vi "Avoid obstacle button2.0.vi"() -> ()   [LabVIEW 2015]
uses:
  <userlib>/KNR OS 3.0 LabVIEW Toolkit/Type Definition/Resource.ctl
  <userlib>/KNR OS 3.0 LabVIEW Toolkit/Type Definition/DC Motor Port.ctl
  <userlib>/KNR OS 3.0 LabVIEW Toolkit/Type Definition/Ultrasonic Port Number.ctl
  <vilib>/myRIO/Common/Instrument Driver Framework/myRIO v1.0/UART/vis/myRIO v1.0 Close UART.vi
  <vilib>/myRIO/Common/Instrument Driver Framework/Utilities/vis/FPGA Ref Manager.vi
  <vilib>/myRIO/Common/Instrument Driver Framework/myRIO v1.0/myRIO v1.0 Reset FPGA.vi
  <vilib>/myRIO/Common/Instrument Driver Framework/myRIO v1.0/IRQ/vis/myRIO v1.0 IRQ Info FGV.vi
  <vilib>/myRIO/Common/Instrument Driver Framework/myRIO v1.0/IRQ/vis/myRIO v1.0 Timer IRQ Info FGV.vi
  <vilib>/myRIO/Common/Instrument Driver Framework/myRIO v1.0/IRQ/vis/myRIO v1.0 ISR Agent.vi
  <vilib>/myRIO/Instrument Drivers/Utilities/Utilities.lvlib
panel:
  in  "stop":bool
  in  "forward speed":dbl=5.8 format="%#_13g"
  out "Speed R 2":dbl=4.06
  out "Speed L 2":dbl=4.06
  in  "upper limit r":dbl=9.0
  in  "upper limit l":dbl=10.0
  in  "Speed":dbl=8.0
  in  "Distance":dbl=35.0
  in  "Kp":dbl=0.3
  in  "Reverse Encoder R":bool=TRUE
  in  "Reverse Encoder L":bool
  in  "Y":dbl
  in  "X":dbl=190.0
  out "Pos R":dbl=170.41358455446547
  out "Pos L":dbl=162.57741982327175
  out "Actual X":dbl=165.0804505801855
  out "Actual Y":dbl=-0.734330747670838
  out "Theta":dbl=21.37996031746032 caption="Heading"
  in  "Reset Encoder R":bool
  in  "Reset Encoder L":bool
  in  "L set Us":dbl=50.0 format="%#_13g"
  in  "Mid set IR":dbl=46.0 format="%#_13g"
  in  "R set Us":dbl=25.0 format="%#_13g"
  out "Case":dbl
  out "L":dbl(slide)=299.99420158565044 scale=0.0..300.0
  out "mid":dbl(slide)=1010.0268999999998 scale=0.0..300.0
  out "R":dbl(slide)=262.09784746170044 scale=0.0..300.0
  out "L Us":dbl=299.99420158565044
  out "MID Us":dbl=1010.0268999999998
  out "R Us":dbl=262.09784746170044
  out "Velocity L (cts/s)":dbl=-2062.5
  in  "?":bool
  out "Velocity R (cts/s)":dbl=3750.0
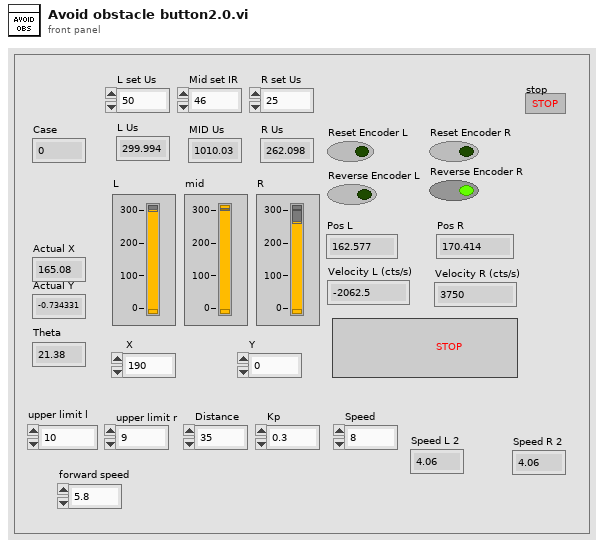
[diagram p1: front panel]
types:
  T1 = typedef "DC Motor Port.ctl" = u16
  T2 = typedef "Resource.ctl" = enum16{"KNRm_DDRC", "KNRm_DDDD", "KNRm_DDDR", "KNRm_DDDC", "KNR"}
  T3 = typedef "KNR3 Reference.ctl" = cluster{"FPGA Session":refnum<class "FPGA Interface Base.lvclass">, "Resource":T2}
  T4 = typedef "Ultrasonic Port Number.ctl" = u16
  T5 = cluster{"Dist 1(cm)":dbl, "Dist 2(cm)":dbl, "Dist 3 (cm)":dbl, "Dist 4 (cm)":dbl}
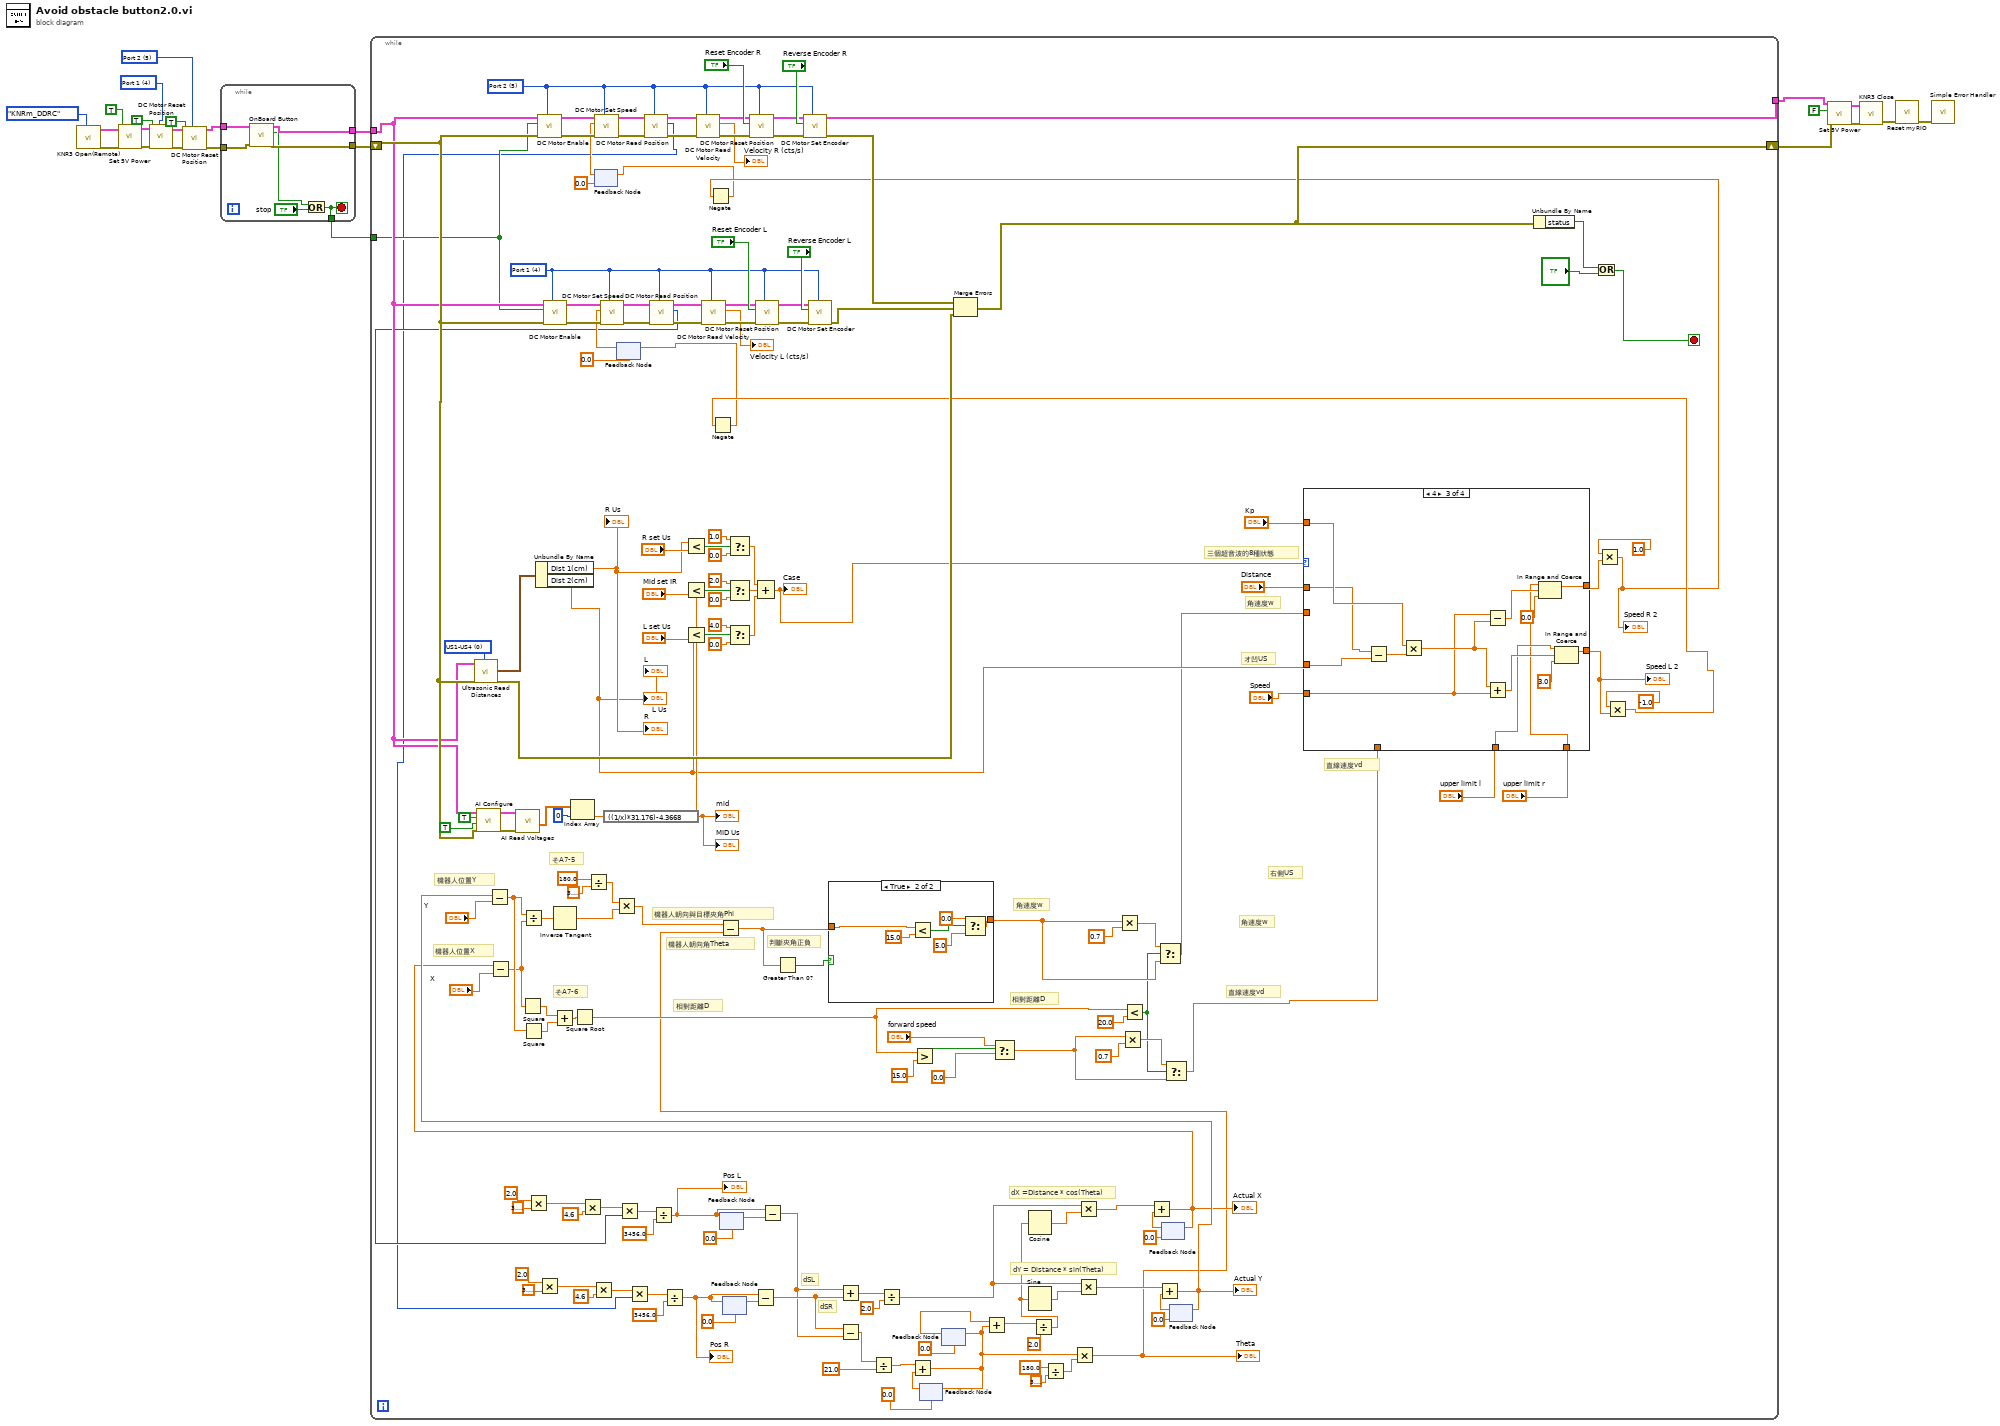
[diagram p0: block diagram]
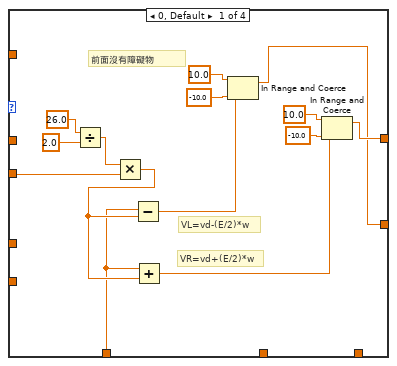
[diagram p2: hidden frame]
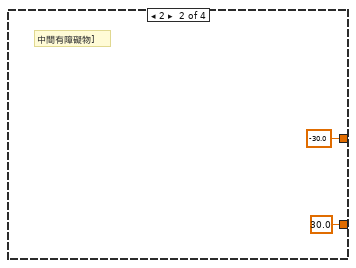
[diagram p3: hidden frame]
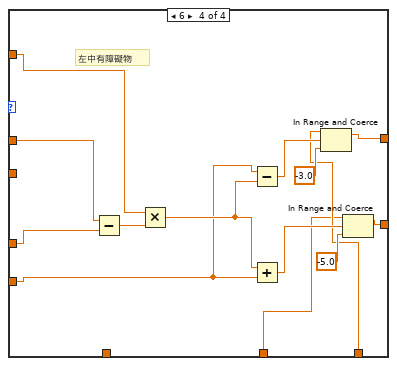
[diagram p4: hidden frame]
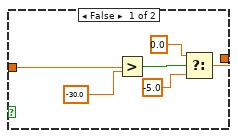
[diagram p5: hidden frame]
diagram:
  w8 = T1 5 items=["Port 1"=4, "Port 2"=5, "Port 3"=6, "Port 4"=7, "Port 5"=8, "Port 6"=9, "Port 7"=10] ("Port Number 2")
  w9 = T1 4 items=["Port 1"=4, "Port 2"=5, "Port 3"=6, "Port 4"=7, "Port 5"=8, "Port 6"=9, "Port 7"=10] ("Port Number")
  n1 = call "KNR3 Open(Remote).vi"("Resource"=Resource."KNRm_DDRC") -> ("error out"=w19:errorcluster, "KNR out"=w20:T3)  [unwired: 9 in]
  n2 = call <userlib>:"Set 5V Power.vi"("error in (no error)"=w19, "5V Power(T)"=TRUE ("5V Power"), "KNR in"=w20) -> ("error out"=w10:errorcluster, "KNR out"=w13:T3)  [unwired: 7 in]
  n3 = call <userlib>:"DC Motor Reset Position.vi"("Port (DS1)"=w9, "error in (no error)"=w10, "Reset(F)"=TRUE, "KNR in"=w13) -> ("error out"=w11:errorcluster, "KNR out"=w12:T3)  [unwired: 6 in]
  n4 = call <userlib>:"DC Motor Reset Position.vi"("Port (DS1)"=w8, "error in (no error)"=w11, "Reset(F)"=TRUE, "KNR in"=w12) -> ("error out"=w4:errorcluster, "KNR out"=w3:T3)  [unwired: 6 in]
  n5 = while {
    tunnel: [w31] -> w5
    tunnel: w4 -> [w30]
    tunnel: w3 -> [w29]
    tunnel: [w28] -> w2
    tunnel: [w25] -> w1
    stop <- w25 stop-if-true
    n6 = call <userlib>:"OnBoard Button.vi"("error in (no error)"=w30, "KNR in"=w29) -> ("error out"=w31:errorcluster, "value"=w27:bool, "KNR out"=w28:T3)  [unwired: 7 in]
    n7 = Or(x=w27, y="stop") -> (x .or. y?=w25:bool)
  }
  n8 = while {
    tunnel: [w190] -> w17
    shift-right: [w173] -> w16
    shift-left: w5 -> [w136]
    tunnel: w2 -> [w43]
    tunnel: w1 -> [w42]
    stop <- w186 stop-if-true
    w172 = T4 0 items=["US1-US4"=0, "US5-US8"=2] ("Port Number")
    w176 = T1 4 items=["Port 1"=4, "Port 2"=5, "Port 3"=6, "Port 4"=7, "Port 5"=8, "Port 6"=9, "Port 7"=10] ("Port Number 2")
    w185 = T1 5 items=["Port 1"=4, "Port 2"=5, "Port 3"=6, "Port 4"=7, "Port 5"=8, "Port 6"=9, "Port 7"=10] ("Port Number")
    # "角速度w"
    # "直線速度vd"
    # "オ凹US"
    # "右側US"
    # "そΑ7-5"
    # "そΑ7-6"
    # "相對距離D"
    # "機器人朝向角Theta"
    # "機器人位置Y"
    # "機器人位置X"
    # "三個超音波的8種狀態"
    # "直線速度vd"
    # "角速度w"
    # "角速度w"
    # "判斷夾角正負"
    # "機器人朝向與目標夾角Phi"
    # "相對距離D"
    # "dSR"
    # "dSL"
    # "dY = Distance * sin(Theta)"
    # "dX =Distance * cos(Theta)"
    n9 = call <userlib>:"Ultrasonic Read Distances.vi"("Port (US1-US4 for KNR)"=w172, "error in (no error)"=w136, "KNR in"=w43) -> ("error out"=w155:errorcluster, "Ultrasonic output"=w171:T5)  [unwired: 6 in, 1 out]
    n10 = call <userlib>:"AI Configure.vi"("error in (no error)"=w136, "8-15 Single ended(T)"=TRUE, "0-7 Single ended(T)"=TRUE, "KNR in"=w43) -> ("error out"=w144:errorcluster, "KNR out"=w143:T3)  [unwired: 6 in]
    n11 = call <userlib>:"AI Read Voltages.vi"("error in (no error)"=w144, "KNR in"=w143) -> ("Voltages"=w139:dbl[])  [unwired: 6 in, 3 out]
    n12 = Multiply(x=2.0, y=3.141592653589793) -> (x*y=w131:dbl)
    n13 = Unbundle By Name(w171) -> ("Dist 1(cm)"=w65:dbl, "Dist 2(cm)"=w61:dbl)
    "R Us" <- w65
    "L Us" <- w61
    "R" <- w65
    "L" <- w61
    n14 = call <userlib>:"DC Motor Enable.vi"("Port (DS1)"=w185, "error in (no error)"=w136, "Enable Motor(F)"=w42, "KNR in"=w43) -> ("error out"=w195:errorcluster, "KNR out"=w154:T3)  [unwired: 6 in]
    n15 = Multiply(x=2.0, y=3.141592653589793) -> (x*y=w124:dbl)
    n16 = call <userlib>:"DC Motor Enable.vi"("Port (DS1)"=w176, "error in (no error)"=w136, "Enable Motor(F)"=w42, "KNR in"=w43) -> ("error out"=w184:errorcluster, "KNR out"=w145:T3)  [unwired: 6 in]
    n17 = Index Array(array=w139, index=0) -> (element=w138:dbl)
    n18 = Multiply(x=w131, y=4.6 ("wheel radius (cm)")) -> (x*y=w129:dbl)
    n19 = Divide(x=180.0, y=3.141592653589793) -> (x/y=w79:dbl)
    n20 = Multiply(x=w124, y=4.6 ("wheel radius (cm)")) -> (x*y=w122:dbl)
    n21 = feedback #1(0.0) -> (w64:dbl)
    n22 = call <userlib>:"DC Motor Set Speed.vi"("Port (DS1)"=w185, "error in (no error)"=w195, "Speed (+-100%)"=w64, "KNR in"=w154) -> ("error out"=w194:errorcluster, "KNR out"=w153:T3)  [unwired: 6 in]
    n23 = expression code="((1/x)*31.176)-4.3668"(w138) -> (w137:dbl)
    "MID Us" <- w137
    "mid" <- w137
    n24 = feedback #2(0.0 ("upper limit L")) -> (w63:dbl)
    n25 = call <userlib>:"DC Motor Set Speed.vi"("Port (DS1)"=w176, "error in (no error)"=w184, "Speed (+-100%)"=w63, "KNR in"=w145) -> ("error out"=w183:errorcluster, "KNR out"=w146:T3)  [unwired: 6 in]
    n26 = call <userlib>:"DC Motor Read Position.vi"("Port (DS1)"=w185, "error in (no error)"=w194, "KNR in"=w153) -> ("error out"=w193:errorcluster, "Position"=w37:i32, "KNR out"=w152:T3)  [unwired: 6 in]
    n27 = Multiply(x=w122, y=w37) -> (x*y=w127:dbl)
    n28 = call <userlib>:"DC Motor Read Position.vi"("Port (DS1)"=w176, "error in (no error)"=w183, "KNR in"=w146) -> ("error out"=w182:errorcluster, "Position"=w38:i32, "KNR out"=w147:T3)  [unwired: 6 in]
    n29 = Multiply(x=w129, y=w38) -> (x*y=w134:dbl)
    n30 = Divide(x=w134, y=3456.0 ("Counts per rev")) -> (x/y=w97:dbl)
    "Pos L" <- w97
    n31 = Divide(x=w127, y=3456.0 ("Counts per rev")) -> (x/y=w98:dbl)
    "Pos R" <- w98
    n32 = Less?(x=w65, y="R set Us") -> (x < y?=w167:bool)
    n33 = Less?(x=w137, y="Mid set IR") -> (x < y?=w166:bool)
    n34 = Less?(x=w61, y="L set Us") -> (x < y?=w165:bool)
    n35 = call <userlib>:"DC Motor Read Velocity.vi"("Port (DS1)"=w185, "error in (no error)"=w193, "KNR in"=w152) -> ("error out"=w192:errorcluster, "Velocity (cts/sec)"=→"Velocity R (cts/s)":dbl, "KNR out"=w151:T3)  [unwired: 6 in]
    n36 = call <userlib>:"DC Motor Read Velocity.vi"("Port (DS1)"=w176, "error in (no error)"=w182, "KNR in"=w147) -> ("error out"=w181:errorcluster, "Velocity (cts/sec)"=→"Velocity L (cts/s)":dbl, "KNR out"=w148:T3)  [unwired: 6 in]
    n37 = feedback #3(0.0 ("Left Wheel Distance")) -> (w112:dbl)
    n38 = feedback-in #3(w97) -> ()
    n39 = feedback #4(0.0 ("Right Wheel Distance")) -> (w111:dbl)
    n40 = feedback-in #4(w98) -> ()
    n41 = Select(t=1.0, s=w167, f=0.0) -> (s? t:f=w157:dbl)
    n42 = Select(t=2.0, s=w166, f=0.0) -> (s? t:f=w158:dbl)
    n43 = Select(t=4.0, s=w165, f=0.0) -> (s? t:f=w156:dbl)
    n44 = call <userlib>:"DC Motor Reset Position.vi"("Port (DS1)"=w185, "error in (no error)"=w192, "Reset(F)"="Reset Encoder R", "KNR in"=w151) -> ("error out"=w191:errorcluster, "KNR out"=w150:T3)  [unwired: 6 in]
    n45 = Subtract(x=w98, y=w111) -> (x-y=w108:dbl)
    n46 = call <userlib>:"DC Motor Reset Position.vi"("Port (DS1)"=w176, "error in (no error)"=w181, "Reset(F)"="Reset Encoder L", "KNR in"=w148) -> ("error out"=w180:errorcluster, "KNR out"=w149:T3)  [unwired: 6 in]
    n47 = Compound Arithmetic op=ADD(w157, w158, w156) -> (w62:dbl)
    "Case" <- w62
    n48 = Subtract(x=w97, y=w112) -> (x-y=w107:dbl)
    n49 = call <userlib>:"DC Motor Set Encoder.vi"("Port (DS1)"=w185, "error in (no error)"=w191, "Reverse?(F)"="Reverse Encoder R", "KNR in"=w150) -> ("error out"=w174:errorcluster, "KNR out"=w190:T3)  [unwired: 6 in]
    n50 = call <userlib>:"DC Motor Set Encoder.vi"("Port (DS1)"=w176, "error in (no error)"=w180, "Reverse?(F)"="Reverse Encoder L", "KNR in"=w149) -> ("error out"=w175:errorcluster)  [unwired: 6 in, 1 out]
    n51 = Subtract(x=w108, y=w107) -> (x-y=w118:dbl)
    n52 = Add(x=w107, y=w108) -> (x+y=w116:dbl)
    n53 = Divide(x=w118, y=21.0 ("Wheel Base")) -> (x/y=w105:dbl)
    n54 = Divide(x=w116, y=2.0) -> (x/y=w114:dbl)
    n55 = feedback #5(0.0) -> (w106:dbl)
    n56 = Add(x=w105, y=w106) -> (x+y=w44:dbl)
    n57 = feedback-in #5(w44) -> ()
    n58 = feedback #6(0.0) -> (w53:dbl)
    n59 = feedback-in #6(w44) -> ()
    n60 = Merge Errors(w174, w175, w155) -> (w173:errorcluster)
    n61 = Add(x=w44, y=w53) -> (x+y=w51:dbl)
    n62 = Divide(x=w51, y=2.0) -> (x/y=w49:dbl)
    n63 = Cosine(x=w49) -> (cos(x)=w119:dbl)
    n64 = Sine(x=w49) -> (sin(x)=w52:dbl)
    n65 = Divide(x=180.0, y=3.141592653589793) -> (x/y=w115:dbl)
    n66 = Multiply(x=w44, y=w115) -> (x*y=w66:dbl)
    "Theta" <- w66
    n67 = Multiply(x=w114, y=w119) -> (x*y=w102:dbl)
    n68 = Multiply(x=w114, y=w52) -> (x*y=w99:dbl)
    n69 = feedback #7(0.0 ("Left Wheel Distance")) -> (w103:dbl)
    n70 = Add(x=w102, y=w103) -> (x+y=w67:dbl)
    "Actual X" <- w67
    n71 = Subtract(x=w67, y="X") -> (x-y=w87:dbl)
    n72 = Square(x=w87) -> (x^2=w86:dbl)
    n73 = feedback-in #7(w67) -> ()
    n74 = feedback #8(0.0 ("Left Wheel Distance")) -> (w100:dbl)
    n75 = Add(x=w99, y=w100) -> (x+y=w68:dbl)
    "Actual Y" <- w68
    n76 = Subtract(x=w68, y="Y") -> (x-y=w88:dbl)
    n77 = Divide(x=w88, y=w87) -> (x/y=w94:dbl)
    n78 = Square(x=w88) -> (x^2=w85:dbl)
    n79 = Add(x=w86, y=w85) -> (x+y=w84:dbl)
    n80 = Inverse Tangent(1:w94) -> (0:w91:dbl)
    n81 = Square Root(x=w84) -> (sqrt(x)=w70:dbl)
    n82 = Multiply(x=w79, y=w91) -> (x*y=w78:dbl)
    n83 = Subtract(x=w78, y=w66) -> (x-y=w89:dbl)
    n84 = Greater Than 0?(x=w89) -> (x > 0?=w90:bool)
    n85 = case shown="True" w90 {
      tunnel: w89 -> [w242 w248]
      tunnel: [w247 w249] -> w74
      frame False {
        n86 = Greater?(x=w242, y=-30.0) -> (0:w246:bool)
        n87 = Select(t=0.0, s=w246, f=-5.0 ("x")) -> (s? t:f=w247:dbl)
      }
      frame True {
        n88 = Less?(x=w248, y=15.0) -> (x < y?=w253:bool)
        n89 = Select(t=0.0, s=w253, f=5.0 ("x")) -> (s? t:f=w249:dbl)
      }
    }
    n90 = Greater?(x=w70, y=15.0) -> (0:w83:bool)
    n91 = Select(t="forward speed", s=w83, f=0.0) -> (s? t:f=w71:dbl)
    n92 = Multiply(x=w74, y=0.7) -> (x*y=w76:dbl)
    n93 = Multiply(x=w71, y=0.7) -> (x*y=w73:dbl)
    n94 = Less?(x=w70, y=20.0) -> (x < y?=w69:bool)
    n95 = Select(t=w76, s=w69, f=w74) -> (s? t:f=w60:dbl)
    n96 = Select(t=w73, s=w69, f=w71) -> (s? t:f=w59:dbl)
    n97 = feedback-in #8(w68) -> ()
    n98 = case shown="4" w62 {
      tunnel: w61 -> [_ _ w221 w233]
      tunnel: [w198 30.0 ("upper limit") w220 w234] -> w32
      tunnel: [w199 -30.0 ("upper limit 2") w219 w235] -> w40
      tunnel: w60 -> [w201 _ _ _]
      tunnel: w59 -> [w200 _ _ _]
      tunnel: "Kp" -> [_ _ w218 w231]
      tunnel: "Distance" -> [_ _ w217 w232]
      tunnel: "Speed" -> [_ _ w216 w230]
      tunnel: "upper limit r" -> [_ _ w214 w229]
      tunnel: "upper limit l" -> [_ _ w215 w228]
      frame 0, Default {
        # "前面沒有障礙物"
        # "VR=vd+(E/2)*w"
        # "VL=vd-(E/2)*w"
        n99 = Divide(x=26.0, y=2.0) -> (x/y=w210:dbl)
        n100 = Multiply(x=w210, y=w201) -> (x*y=w211:dbl)
        n101 = Subtract(x=w200, y=w211) -> (x-y=w205:dbl)
        n102 = Add(x=w200, y=w211) -> (x+y=w202:dbl)
        n103 = In Range and Coerce(upper limit=10.0, x=w205, lower limit=-10.0) -> (coerced(x)=w198:dbl)  [unwired: 1 out]
        n104 = In Range and Coerce(upper limit=10.0, x=w202, lower limit=-10.0) -> (coerced(x)=w199:dbl)  [unwired: 1 out]
      }
      frame 2 {
        # "中間有障礙物]"
      }
      frame 4 {
        n105 = Subtract(x=w217, y=w221) -> (x-y=w227:dbl)
        n106 = Multiply(x=w218, y=w227) -> (x*y=w226:dbl)
        n107 = Subtract(x=w216, y=w226) -> (x-y=w223:dbl)
        n108 = Add(x=w226, y=w216) -> (x+y=w222:dbl)
        n109 = In Range and Coerce(upper limit=w214, x=w223, lower limit=0.0) -> (coerced(x)=w219:dbl)  [unwired: 1 out]
        n110 = In Range and Coerce(upper limit=w215, x=w222, lower limit=3.0) -> (coerced(x)=w220:dbl)  [unwired: 1 out]
      }
      frame 6 {
        # "左中有障礙物"
        n111 = Subtract(x=w232, y=w233) -> (x-y=w241:dbl)
        n112 = Multiply(x=w231, y=w241) -> (x*y=w240:dbl)
        n113 = Subtract(x=w230, y=w240) -> (x-y=w237:dbl)
        n114 = Add(x=w240, y=w230) -> (x+y=w236:dbl)
        n115 = In Range and Coerce(upper limit=w229, x=w237, lower limit=-3.0) -> (coerced(x)=w235:dbl)  [unwired: 1 out]
        n116 = In Range and Coerce(upper limit=w228, x=w236, lower limit=-5.0) -> (coerced(x)=w234:dbl)  [unwired: 1 out]
      }
    }
    "Speed L 2" <- w32
    n117 = Unbundle By Name(w173) -> ("status"=w197:bool)
    n118 = Or(x=w197, y="?") -> (x .or. y?=w186:bool)
    n119 = Multiply(x=1.0 ("upper limit 2"), y=w40) -> (x*y=w34:dbl)
    "Speed R 2" <- w34
    n120 = Negate(x=w34) -> (-x=w33:dbl)
    n121 = feedback-in #1(w33) -> ()
    n122 = Multiply(x=-1.0 ("upper limit 2"), y=w32) -> (x*y=w36:dbl)
    n123 = Negate(x=w36) -> (-x=w35:dbl)
    n124 = feedback-in #2(w35) -> ()
  }
  n125 = call <userlib>:"Set 5V Power.vi"("error in (no error)"=w16, "5V Power(T)"=FALSE ("5V Power"), "KNR in"=w17) -> ("error out"=w23:errorcluster, "KNR out"=w21:T3)  [unwired: 7 in]
  n126 = call <userlib>:"KNR3 Close.vi"("error in (no error)"=w23, "KNR in"=w21) -> ("error out"=w15:errorcluster)  [unwired: 9 in]
  n127 = call <vilib>:"Reset myRIO.vi"("error in (no error)"=w15) -> ("error out"=w14:errorcluster)  [unwired: 10 in]
  n128 = call <vilib>:"Simple Error Handler.vi"("error in (no error)"=w14) -> ()  [unwired: 4 in, 5 out]
